vi "CloseMark10Monitor.vi"(8 "Error In":errorcluster) -> (0 "Error Out":errorcluster)   [LabVIEW 2019, in "Mark 10 TSTM-DC.lvlib" / "Mark 10 Event Monitor.lvlib"]
uses:
  Mark 10 Event Monitor.lvlib
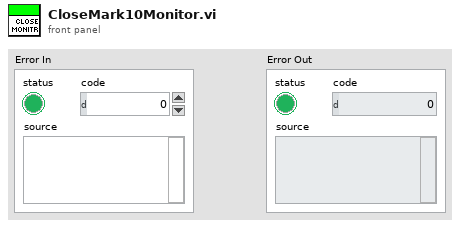
[diagram p1: front panel]
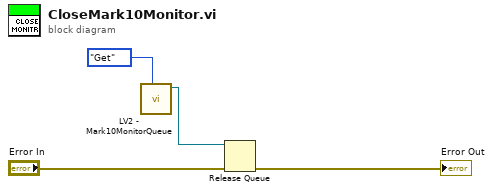
[diagram p0: block diagram]
diagram:
  n1 = call "LV2 - Mark10MonitorQueue.vi"("Enum"=enum16{"Set", "Get"}."Get") -> ("Mark10Monitor out"=w1:refnum<queue>)  [unwired: 10 in]
  n2 = Release Queue(queue=w1, error in (no error)="Error In") -> (error out=→"Error Out":errorcluster)  [unwired: 1 in, 2 out]
